vi "SW_Generate_Segmented_Plot.vi"(0 "Zones Display input":picture, 1 "Amount of border segments":u8=8, 2 "Amount of midfield segments":u8=4, 3 "Border segments starting angle":i16(knob) min=-180 max=180 scale=-180.0..180.0, 4 "Midfield segments starting angle":i16(knob) min=-180 max=180 scale=-180.0..180.0, 5 "Error In":errorcluster, 6 "Diameter of the cage, mm":u16(knob)=180 scale=20.0..250.0, 7 "Midfield segments outer radius, mm":i16(knob)=60 min=-180 max=180 scale=0.0..90.0, 8 "R-gap between segments, mm":u8=10, 9 "Center segment outer radius, mm":i16(knob)=30 min=-180 max=180 scale=0.0..90.0, 16 "Colors array for outer segments":u32[](array[numeric])=[14102567, 16625249, 14742520, 7646673, 16018755, 16703632, 11262441, 4552116], 17 "Colors array for midfield segments":u32[](array[numeric])=[8073876, 10935200, 34871, 12756431], 18 "Color for central segment":u32=16777113) -> (14 "Zones Display output":picture, 15 "Pixels per mm":dbl=2.533333333333333, 19 "Error Out":errorcluster)   [LabVIEW 2016]
panel:
  out "Radius of displayed outer segments, pix":dbl=228.0
  in  "Amount of central segments":u8=1
  in  "Background color":u32(colorbox)=13816530
  out "Draw Area Size":cluster{"Width":dbl, "Height":dbl}={"Width"=480.0, "Height"=480.0}
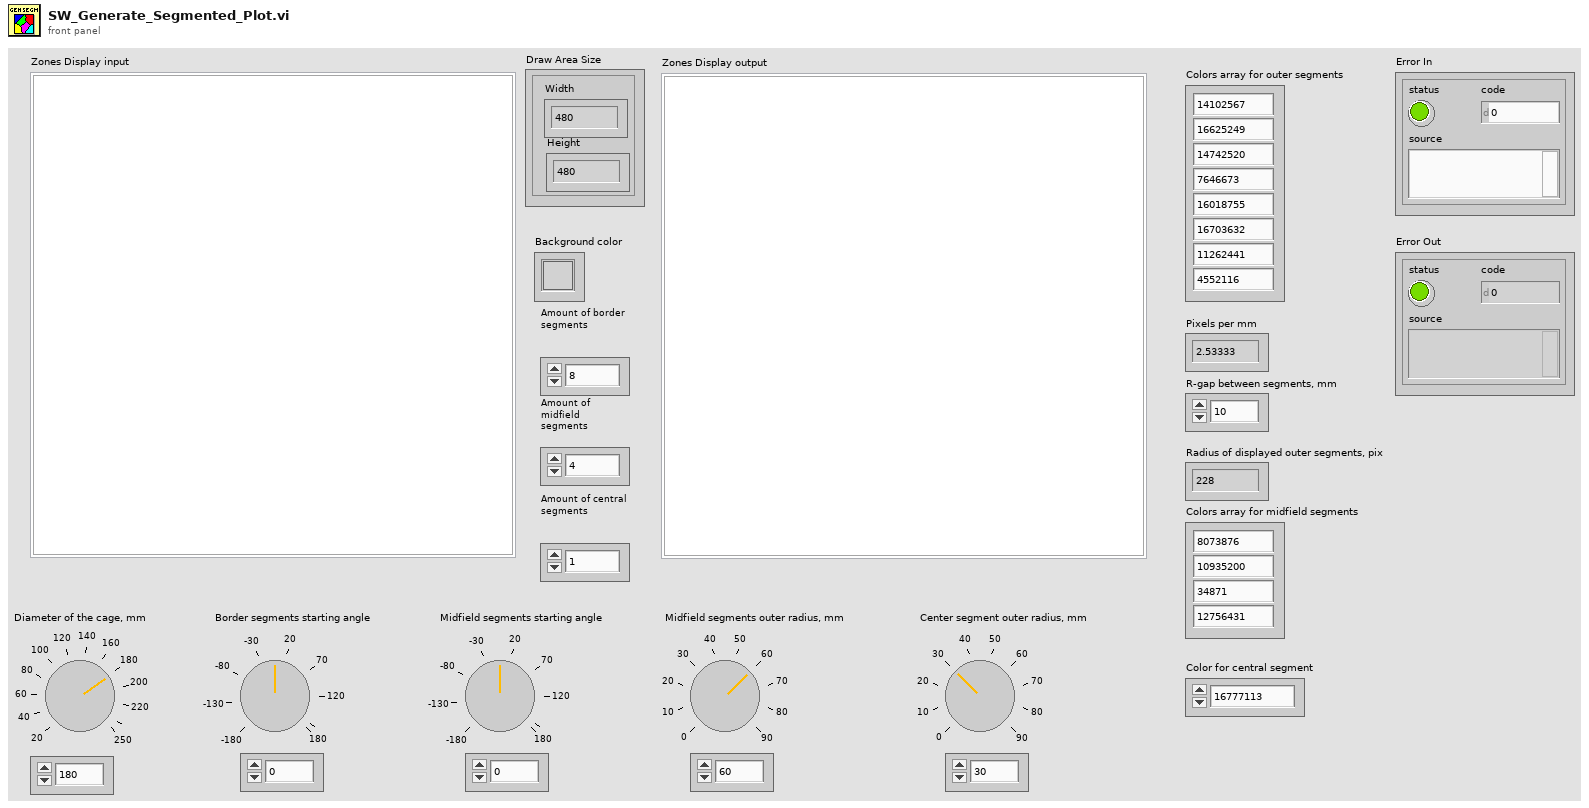
[diagram p1: front panel]
types:
  T1 = cluster{"Width":u16, "Style":enum32{"Solid", "Dash", "Dot", "DashDot", "DashDotDot"}}
  T2 = typedef "LVBoundsTypeDef.ctl" = cluster{"Width":u32, "Height":u32}
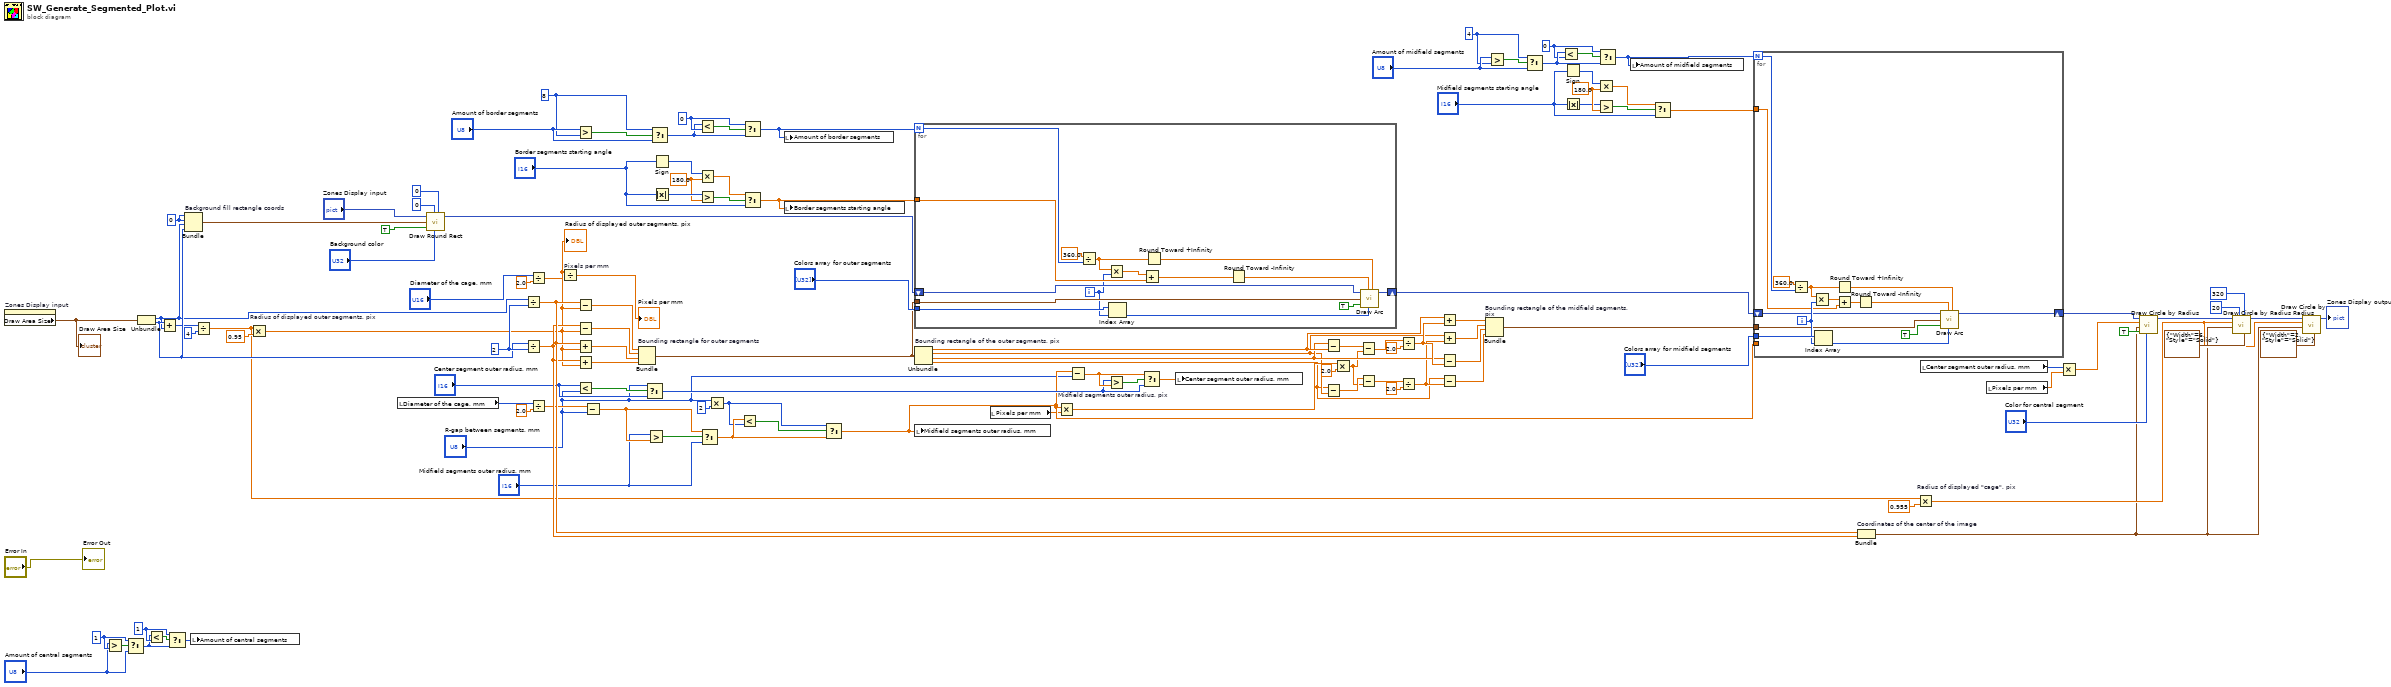
[diagram p0: block diagram]
diagram:
  w57 = 180.0 ("y")
  w65 = u8 1 ("y")
  w62 = u8 1 ("y")
  w67 = u8 4 ("y")
  w71 = u8 0 ("y")
  w98 = u8 0 ("y")
  w100 = u8 8 ("y")
  w104 = 180.0 ("y")
  w115 = u32 2 ("y")
  w117 = 0
  n1 = property on="Zones Display input" class="Pict"() -> ("Draw Area Size"=w118:T2)  [unwired: 2 in, 2 out]
  "Draw Area Size" <- w118
  n2 = Greater?(x="Amount of central segments", y=w65) -> (0:w64:bool)
  n3 = Select(t=w65, s=w64, f="Amount of central segments") -> (s? t:f=w61:u8)
  n4 = Unbundle(w118) -> ("Width"=w113:u32, "Height"=w114:u32)
  n5 = Less?(x=w61, y=w62) -> (x < y?=w63:bool)
  n6 = Add(x=w114, y=w113) -> (x+y=w112:u32)
  n7 = Select(t=w62, s=w63, f=w61) -> (s? t:f=w59:u8)
  n8 = Bundle "Background fill rectangle coords"(w117, w117, "Width"=w113, "Height"=w114) -> (w94:cluster{i32, i32, "Width":u32, "Height":u32})  [unwired: 1 in]
  n9 = local write "Amount of central segments"(w59) -> ()
  n10 = Divide(x=w112, y=u32 4) -> (x/y=w77:dbl)
  n11 = Multiply "Radius of displayed outer segments, pix"(x=w77, y=0.95) -> (x*y=w83:dbl)
  "Radius of displayed outer segments, pix" <- w83
  n12 = local read "Diameter of the cage, mm"() -> (w51:u16)
  n13 = call <vilib>:"Draw Round Rect.vi"("picture"="Zones Display input", "oval width"=i16 0, "rect"=w94, "fill?(F)"=TRUE, "color(black)"="Background color", "oval height"=i16 0) -> ("new picture"=w93:picture)  [unwired: 3 in]
  n14 = Divide(x=w113, y=w115) -> (x/y=w92:dbl)
  n15 = Divide(x=w114, y=w115) -> (x/y=w91:dbl)
  n16 = Divide(x="Diameter of the cage, mm", y=2.0) -> (x/y=w75:dbl)
  n17 = Divide(x=w51, y=2.0) -> (x/y=w45:dbl)
  n18 = Divide "Pixels per mm"(x=w83, y=w75) -> (x/y=→"Pixels per mm":dbl)
  n19 = Greater?(x="Amount of border segments", y=w100) -> (0:w102:bool)
  n20 = Subtract(x=w92, y=w83) -> (x-y=w90:dbl)
  n21 = Subtract(x=w91, y=w83) -> (x-y=w89:dbl)
  n22 = Add(x=w92, y=w83) -> (x+y=w88:dbl)
  n23 = Add(x=w91, y=w83) -> (x+y=w87:dbl)
  n24 = Less?(x="Center segment outer radius, mm", y="R-gap between segments, mm") -> (x < y?=w43:bool)
  n25 = Subtract(x=w45, y="R-gap between segments, mm") -> (x-y=w49:dbl)
  n26 = Bundle "Bounding rectangle for outer segments"(w90, w89, w88, w87) -> (w35:cluster{dbl, dbl, dbl, dbl})  [unwired: 1 in]
  n27 = Select(t="R-gap between segments, mm", s=w43, f="Center segment outer radius, mm") -> (s? t:f=w39:i16)
  n28 = Greater?(x="Midfield segments outer radius, mm", y=w49) -> (0:w50:bool)
  n29 = Select(t=w100, s=w102, f="Amount of border segments") -> (s? t:f=w97:u8)
  n30 = Sign(1:"Border segments starting angle") -> (0:w105:i16)
  n31 = Absolute Value(x="Border segments starting angle") -> (abs(x)=w108:i16)
  n32 = Less?(x=w97, y=w98) -> (x < y?=w99:bool)
  n33 = Multiply(x=w105, y=w104) -> (x*y=w103:dbl)
  n34 = Greater?(x=w108, y=w104) -> (0:w107:bool)
  n35 = Select(t=w49, s=w50, f="Midfield segments outer radius, mm") -> (s? t:f=w46:dbl)
  n36 = Multiply(x="R-gap between segments, mm", y=u8 2) -> (x*y=w37:u8)
  n37 = Less?(x=w46, y=w37) -> (x < y?=w47:bool)
  n38 = Select(t=w98, s=w99, f=w97) -> (s? t:f=w96:u8)
  n39 = Select(t=w103, s=w107, f="Border segments starting angle") -> (s? t:f=w95:dbl)
  n40 = local write "Amount of border segments"(w96) -> ()
  n41 = local write "Border segments starting angle"(w95) -> ()
  n42 = Select(t=w37, s=w47, f=w46) -> (s? t:f=w34:dbl)
  n43 = for {
    N: w96 -> [w132]
    tunnel: w95 -> [w130]
    shift-right: [w136] -> w73
    shift-left: w93 -> [w135]
    tunnel: w35 -> [w134]
    tunnel: "Colors array for outer segments" -> [w126]
    i -> [w125]
    n44 = Divide(x=360.0, y=w132) -> (x/y=w133:dbl)
    n45 = Multiply(x=w133, y=w125) -> (x*y=w131:dbl)
    n46 = Index Array(array=w126, index=w125) -> (element=w124:u32)
    n47 = Add(x=w131, y=w130) -> (x+y=w129:dbl)
    n48 = Round Toward +Infinity(x=w133) -> (ceil(x): smallest int >= x=w128:dbl)
    n49 = Round Toward -Infinity(1:w129) -> (0:w127:dbl)
    n50 = call <vilib>:"Draw Arc.vi"("picture"=w135, "start angle[degrees]"=w127, "rect"=w134, "fill?(F)"=TRUE, "color(black)"=w124, "arc size[degrees]"=w128) -> ("new picture"=w136:picture)  [unwired: 3 in]
  }
  n51 = Unbundle "Bounding rectangle of the outer segments, pix"(w35) -> (w27:dbl, w19:dbl, w25:dbl, w18:dbl)
  n52 = local write "Midfield segments outer radius, mm"(w34) -> ()
  n53 = local read "Pixels per mm"() -> (w33:dbl)
  n54 = Multiply "Midfield segments outer radius, pix"(x=w34, y=w33) -> (x*y=w31:dbl)
  n55 = Subtract(x=w34, y="R-gap between segments, mm") -> (x-y=w40:dbl)
  n56 = Greater?(x=w39, y=w40) -> (0:w41:bool)
  n57 = Select(t=w40, s=w41, f=w39) -> (s? t:f=w38:dbl)
  n58 = local write "Center segment outer radius, mm"(w38) -> ()
  n59 = Subtract(x=w25, y=w27) -> (x-y=w32:dbl)
  n60 = Subtract(x=w18, y=w19) -> (x-y=w24:dbl)
  n61 = Multiply(x=w31, y=2.0) -> (x*y=w23:dbl)
  n62 = Subtract(x=w32, y=w23) -> (x-y=w29:dbl)
  n63 = Subtract(x=w24, y=w23) -> (x-y=w21:dbl)
  n64 = Divide(x=w29, y=2.0) -> (x/y=w26:dbl)
  n65 = Divide(x=w21, y=2.0) -> (x/y=w20:dbl)
  n66 = Add(x=w27, y=w26) -> (x+y=w17:dbl)
  n67 = Add(x=w19, y=w20) -> (x+y=w14:dbl)
  n68 = Subtract(x=w25, y=w26) -> (x-y=w15:dbl)
  n69 = Subtract(x=w18, y=w20) -> (x-y=w13:dbl)
  n70 = Bundle "Bounding rectangle of the midfield segments, pix"(w17, w14, w15, w13) -> (w16:cluster{dbl, dbl, dbl, dbl})  [unwired: 1 in]
  n71 = Greater?(x="Amount of midfield segments", y=w67) -> (0:w69:bool)
  n72 = Select(t=w67, s=w69, f="Amount of midfield segments") -> (s? t:f=w72:u8)
  n73 = Less?(x=w72, y=w71) -> (x < y?=w70:bool)
  n74 = Sign(1:"Midfield segments starting angle") -> (0:w56:i16)
  n75 = Absolute Value(x="Midfield segments starting angle") -> (abs(x)=w54:i16)
  n76 = Multiply(x=w56, y=w57) -> (x*y=w58:dbl)
  n77 = Greater?(x=w54, y=w57) -> (0:w55:bool)
  n78 = Select(t=w71, s=w70, f=w72) -> (s? t:f=w66:u8)
  n79 = local write "Amount of midfield segments"(w66) -> ()
  n80 = Select(t=w58, s=w55, f="Midfield segments starting angle") -> (s? t:f=w52:dbl)
  n81 = for {
    N: w66 -> [w143]
    shift-right: [w138] -> w9
    shift-left: w73 -> [w139]
    tunnel: w52 -> [w141]
    tunnel: w34 -> [_]
    tunnel: w16 -> [w140]
    tunnel: "Colors array for midfield segments" -> [w145]
    i -> [w142]
    n82 = Divide(x=360.0, y=w143) -> (x/y=w147:dbl)
    n83 = Multiply(x=w147, y=w142) -> (x*y=w148:dbl)
    n84 = Index Array(array=w145, index=w142) -> (element=w144:u32)
    n85 = Round Toward +Infinity(x=w147) -> (ceil(x): smallest int >= x=w150:dbl)
    n86 = Add(x=w148, y=w141) -> (x+y=w149:dbl)
    n87 = Round Toward -Infinity(1:w149) -> (0:w151:dbl)
    n88 = call <vilib>:"Draw Arc.vi"("picture"=w139, "start angle[degrees]"=w151, "rect"=w140, "fill?(F)"=TRUE, "color(black)"=w144, "arc size[degrees]"=w150) -> ("new picture"=w138:picture)  [unwired: 3 in]
  }
  n89 = Bundle "Coordinates of the center of the image"(w92, w91) -> (w2:cluster{dbl, dbl})  [unwired: 1 in]
  n90 = Multiply "Radius of displayed \"cage\", pix"(x=w77, y=0.955) -> (x*y=w78:dbl)
  n91 = local read "Center segment outer radius, mm"() -> (w5:i16)
  n92 = local read "Pixels per mm"() -> (w4:dbl)
  n93 = Multiply(x=w5, y=w4) -> (x*y=w3:dbl)
  n94 = call <vilib>:"Draw Circle by Radius.vi"("color(black)"="Color for central segment", "fill?(F)"=TRUE, "pixel center"=w2, "radius"=w3, "picture"=w9) -> ("new picture"=w8:picture)  [unwired: 6 in]
  n95 = call <vilib>:"Draw Circle by Radius.vi"("pen"=T1 {"Width"=6, "Style"=enum."Solid"}, "arc size(360)"=i16 320, "start angle(0)"=i16 20, "pixel center"=w2, "radius"=w78, "picture"=w8) -> ("new picture"=w85:picture)  [unwired: 5 in]
  n96 = call <vilib>:"Draw Circle by Radius.vi"("pen"=T1 {"Width"=2, "Style"=enum."Solid"}, "pixel center"=w2, "radius"=w78, "picture"=w85) -> ("new picture"=→"Zones Display output":picture)  [unwired: 7 in]
  "Error Out" <- "Error In"
